vi "Stable.vi"(5 "slope/mean thresh":dbl, 7 "std/mean thresh":dbl, 9 "New data point":dbl, 10 "Number of points":dbl, 11 "Array in":dbl[](array[numeric])) -> (2 "Stable?":bool, 3 "Array out":dbl[](array[numeric]))   [LabVIEW 2023]
uses:
  <vilib>/Analysis/1siggen.llb/Ramp Pattern by Delta.vi
  <vilib>/Analysis/NI_AALPro.lvlib
  <vilib>/Analysis/NI_AALBase.lvlib
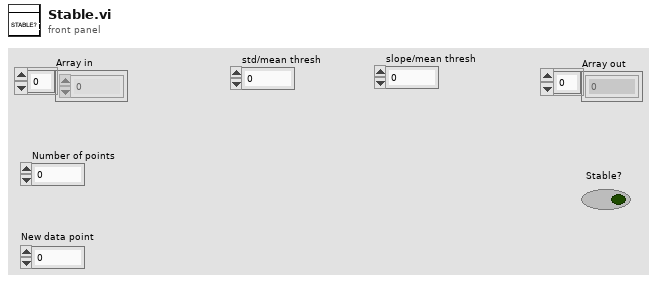
[diagram p1: front panel]
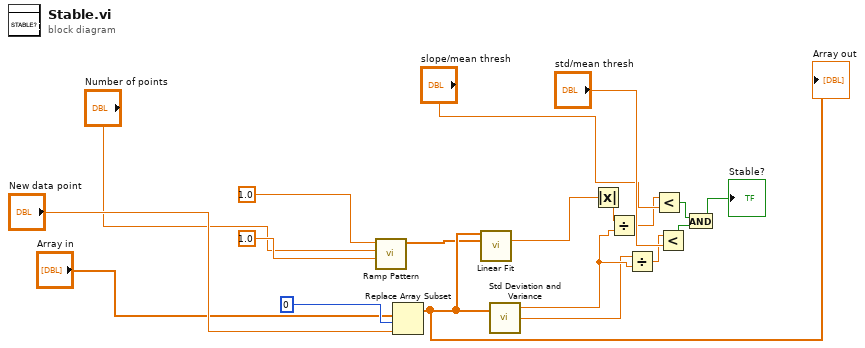
[diagram p0: block diagram]
diagram:
  n1 = call-poly <vilib>:"Ramp Pattern.vi"("start"=1.0, "end"="Number of points", "delta"=1.0) -> ("Ramp Pattern"=w6:dbl[])  [unwired: 6 in, 2 out]
  n2 = Replace Array Subset(array="Array in", new element="New data point", index=0 ("Index")) -> (w8:dbl[])
  "Array out" <- w8
  n3 = call <vilib>:"Linear Fit.vi"("Y"=w8, "X"=w6) -> ("slope"=w7:dbl)  [unwired: 9 in, 4 out]
  n4 = call <vilib>:"Std Deviation and Variance.vi"("X"=w8) -> ("mean"=w14:dbl, "standard deviation"=w13:dbl)  [unwired: 1 in, 1 out]
  n5 = Absolute Value(x=w7) -> (abs(x)=w10:dbl)
  n6 = Divide(x=w10, y=w14) -> (x/y=w11:dbl)
  n7 = Divide(x=w13, y=w14) -> (x/y=w15:dbl)
  n8 = Less?(x=w11, y="slope/mean thresh") -> (x < y?=w18:bool)
  n9 = Less?(x=w15, y="std/mean thresh") -> (x < y?=w17:bool)
  n10 = And(x=w18, y=w17) -> (x .and. y?=→"Stable?":bool)
